vi "PH_4_Pos_Selector.Picture PA Serrated Apperture.vi"(1 "Current Position":T1 items=["unknown", "Position I", "Position II", "Position III", "Position IV", "moving"]) -> (0 "PA Seratted Apperture Array":picture[](array[picture]))   [LabVIEW 2014, in "PH_4_Pos_Selector.lvlib"]
uses:
  PH_4_Pos_Selector.lvlib
  PH_4_Pos_Selector.Position Selector.ctl
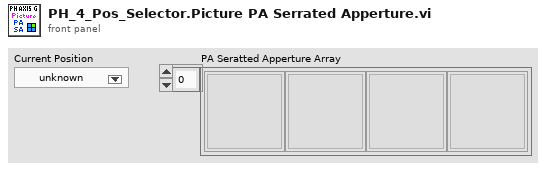
[diagram p1: front panel]
types:
  T1 = typedef "PH_4_Pos_Selector.lvlib/PH_4_Pos_Selector.Position Selector.ctl" = u16
  T2 = cluster{"left":i16, "top":i16, "right":i16, "bottom":i16}[]
  T3 = cluster{"left":i16, "top":i16, "right":i16, "bottom":i16}
  T4 = cluster{"horizontal":enum16{"left", "center", "right"}, "vertical":enum16{"top", "center", "bottom"}}
  T5 = enum16{"User-specified Font", "Application Font", "System Font", "Dialog Font"}
  T6 = cluster{"Font Name:":string, "Size":i16, "Strikeout?":bool, "Italic?":bool, "Underline?":bool, "Outline?":bool, "Shadow?":bool, "Bold?":bool}
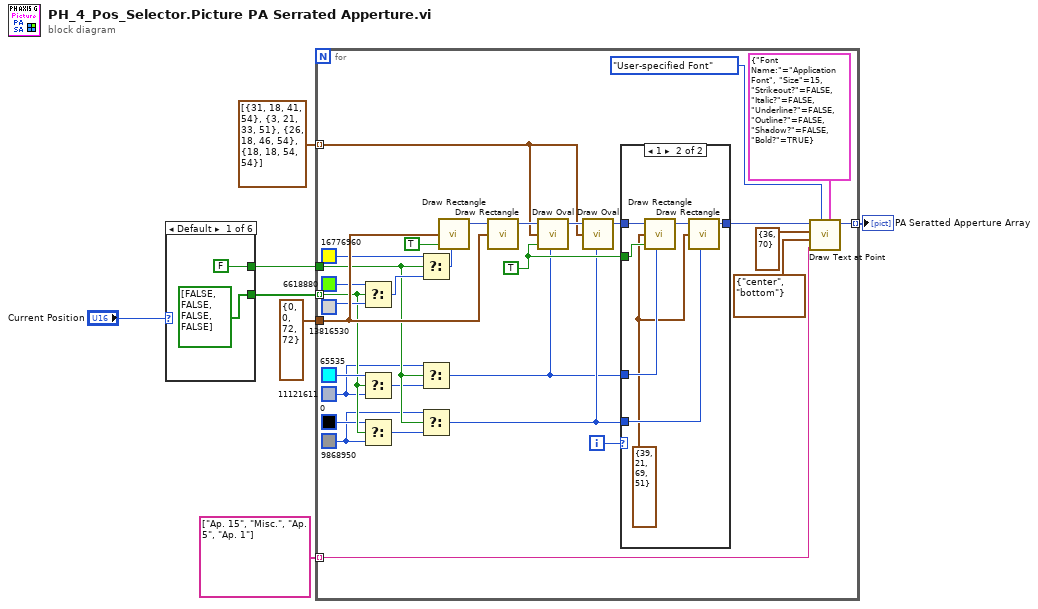
[diagram p0: block diagram]
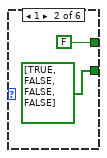
[diagram p2: hidden frame]
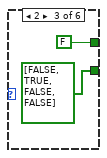
[diagram p3: hidden frame]
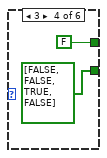
[diagram p4: hidden frame]
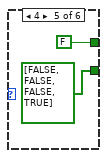
[diagram p5: hidden frame]
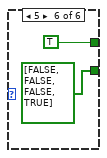
[diagram p6: hidden frame]
diagram:
  n1 = case shown="Default" "Current Position" {
    tunnel: [bool[] [FALSE, FALSE, FALSE, FALSE] bool[] [TRUE, FALSE, FALSE, FALSE] bool[] [FALSE, TRUE, FALSE, FALSE] bool[] [FALSE, FALSE, TRUE, FALSE] bool[] [FALSE, FALSE, FALSE, TRUE] bool[] [FALSE, FALSE, FALSE, TRUE]] -> w6
    tunnel: [FALSE FALSE FALSE FALSE FALSE TRUE] -> w5
    frame Default {
    }
    frame 1 {
    }
    frame 2 {
    }
    frame 3 {
    }
    frame 4 {
    }
    frame 5 {
    }
  }
  n2 = for {
    tunnel: T3 {"left"=0, "top"=0, "right"=72, "bottom"=72} ("rect") -> [w49]
    tunnel: w6 -> [w35] mode=indexing
    tunnel: w5 -> [w26]
    tunnel: [w41] -> w2 mode=indexing
    tunnel: string[] ["Ap. 15", "Misc.", "Ap. 5", "Ap. 1"] -> [w42] mode=indexing
    tunnel: T2 [{"left"=31, "top"=18, "right"=41, "bottom"=54}, {"left"=3, "top"=21, "right"=33, "bottom"=51}, {"left"=26, "top"=18, "right"=46, "bottom"=54}, {"left"=18, "top"=18, "right"=54, "bottom"=54}] -> [w34] mode=indexing
    i -> [w27]
    w28 = TRUE ("fill?(F)")
    w24 = u32 9868950
    w25 = u32 11121611
    n3 = Select(t=u32 6618880, s=w35, f=u32 13816530) -> (s? t:f=w45:u32)
    n4 = Select(t=u32 65535 ("color(black)"), s=w35, f=w25) -> (s? t:f=w21:u32)
    n5 = Select(t=u32 0, s=w35, f=w24) -> (s? t:f=w23:u32)
    n6 = Select(t=u32 16776960, s=w26, f=w45) -> (s? t:f=w44:u32)
    n7 = Select(t=w25, s=w26, f=w21) -> (s? t:f=w20:u32)
    n8 = Select(t=w24, s=w26, f=w23) -> (s? t:f=w22:u32)
    n9 = call <vilib>:"Draw Rectangle.vi"("rect"=w49, "fill?(F)"=TRUE, "color(black)"=w44) -> ("new picture"=w50:picture)  [unwired: 6 in]
    n10 = call <vilib>:"Draw Rectangle.vi"("picture"=w50, "rect"=w49) -> ("new picture"=w39:picture)  [unwired: 7 in]
    n11 = call <vilib>:"Draw Oval.vi"("picture"=w39, "rect"=w34, "fill?(F)"=w28, "color(black)"=w20) -> ("new picture"=w38:picture)  [unwired: 5 in]
    n12 = call <vilib>:"Draw Oval.vi"("picture"=w38, "rect"=w34, "color(black)"=w22) -> ("new picture"=w30:picture)  [unwired: 6 in]
    n13 = case shown="1" w27 {
      tunnel: w30 -> [w51 w57]
      tunnel: [w51 w56] -> w29
      tunnel: w20 -> [_ w55]
      tunnel: w22 -> [_ w54]
      tunnel: w28 -> [_ w53]
      frame Default {
      }
      frame 1 {
        w52 = T3 {"left"=39, "top"=21, "right"=69, "bottom"=51} ("rect")
        n14 = call <vilib>:"Draw Rectangle.vi"("picture"=w57, "rect"=w52, "fill?(F)"=w53, "color(black)"=w55) -> ("new picture"=w58:picture)  [unwired: 5 in]
        n15 = call <vilib>:"Draw Rectangle.vi"("picture"=w58, "rect"=w52, "color(black)"=w54) -> ("new picture"=w56:picture)  [unwired: 6 in]
      }
    }
    n16 = call <vilib>:"Draw Text at Point.vi"("[user-specified font]"=T6 {"Font Name:"="Application Font", "Size"=15, "Strikeout?"=FALSE, "Italic?"=FALSE, "Underline?"=FALSE, "Outline?"=FALSE, "Shadow?"=FALSE, "Bold?"=TRUE}, "desired font(Application)"=T5."User-specified Font", "text"=w42, "alignment(left, top)"=T4 {"horizontal"=enum."center", "vertical"=enum."bottom"}, "origin"=cluster{"x":i32, "y":i32} {"x"=36, "y"=70}, "picture"=w29) -> ("new picture"=w41:picture)  [unwired: 4 in, 1 out]
  }
  "PA Seratted Apperture Array" <- w2
